vi "Com _Grant Right.vi"(6 "UserNo":string, 7 "Command":string, 8 "error in (no error)":errorcluster caption="错误输入（无错误）", 9 "FunctionID":i32, 10 "RoleID":i32, 11 "Traceability 引用句柄":refnum<k24>) -> (0 "error out":errorcluster caption="错误输出", 2 "Com_GrantRight":bool, 3 "Traceability 引用句柄输出":refnum<k24>)   [LabVIEW 2014, in "Traceability.lvlib"]
uses:
  D:/webservice/Traceability.dll
  Traceability.dll
  Traceability.lvlib
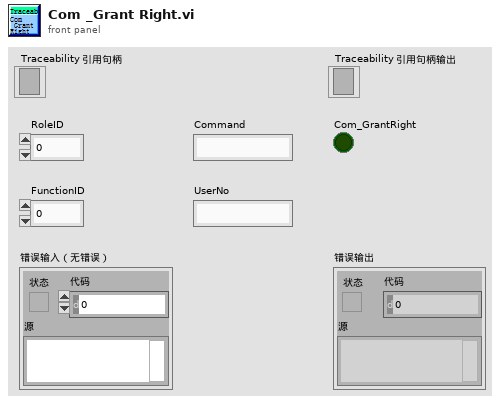
[diagram p1: front panel]
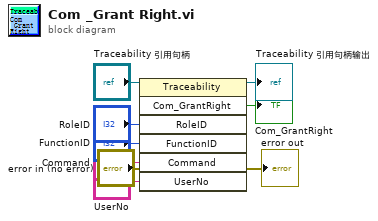
[diagram p0: block diagram]
diagram:
  n1 = invoke class="Traceability" method="Com_GrantRight"(reference="Traceability 引用句柄", error in="error in (no error)", "RoleID"="RoleID", "FunctionID"="FunctionID", "Command"="Command", "UserNo"="UserNo") -> (reference out=→"Traceability 引用句柄输出":refnum<k24>, error out=→"error out":errorcluster, "Com_GrantRight"=→"Com_GrantRight":bool)  [unwired: 1 in, 4 out]
